vi "Test Log.vi"(7 "Name":string="Test Log", 11 "Message":string) -> (3 "BT.lvlib:abs_Node.lvclass":refnum<class "abs_Node.lvclass">)   [LabVIEW 2021]
uses:
  Source/Support/Nodes/abs_Node/abs_Node.lvclass
  Test Log.lvclass
  C:/Users/Tim/Documents/GitHub/LV_Behaviour_Tree/Source/Support/abs_Log/abs_Log.lvclass
  C:/Program Files (x86)/National Instruments/LabVIEW 2021/vi.lib/TSA/Abstract Data Classes/Abs_Types/Type/Abs_Type.lvclass
  C:/Users/Tim/Documents/GitHub/LV_Behaviour_Tree/Source/Support/abs_Node/abs_Node.lvclass
  Source/Support/Nodes/Leaves/abs_Log/abs_Log.lvclass/abs_Log.ctl
  <vilib>/TSA/Abstract Data Classes/Abs_Types/Type/Abs_Type.lvclass/Abs_Type.ctl
  Source/Support/Nodes/Leaves/abs_Log/Properties/Write Message.vi
  <vilib>/TSA/Abstract Data Classes/Abs_Types/Type/Properties/Write Name.vi
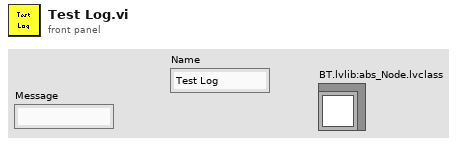
[diagram p1: front panel]
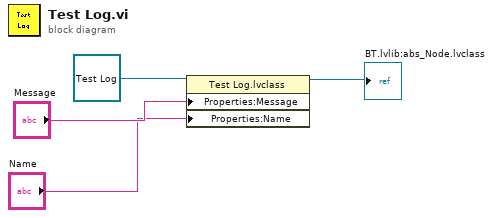
[diagram p0: block diagram]
diagram:
  n1 = property class="Test Log.lvclass"(reference=refnum<class "Test Log.lvclass"> refnum ("Test Log.lvclass"), "Properties:Message"="Message", "Properties:Name"="Name") -> (reference out=→"BT.lvlib:abs_Node.lvclass":refnum<class "Test Log.lvclass">)  [unwired: 1 in, 1 out]
